vi "Calculate Hold-In Voltage Measurements.vi"(0 "Stage Voltage Section":dbl[](array[numeric]), 5 "Stage.Dwell.Level":dbl, 7 "Active Edge":bool) -> (4 "Max Stage":dbl, 6 "Min Stage":dbl, 10 "Avg Max Stage":dbl, 15 "Avg Min Stage":dbl)   [LabVIEW 2019, in "Fuel Injector Analysis Addon Engine.lvlib"]
uses:
  Fuel Injector Analysis Addon Engine.lvlib
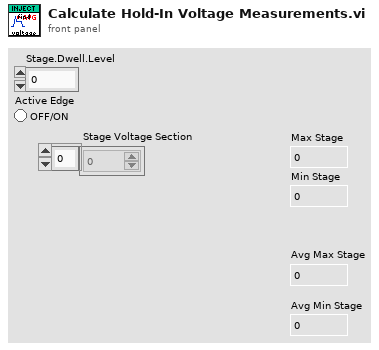
[diagram p1: front panel]
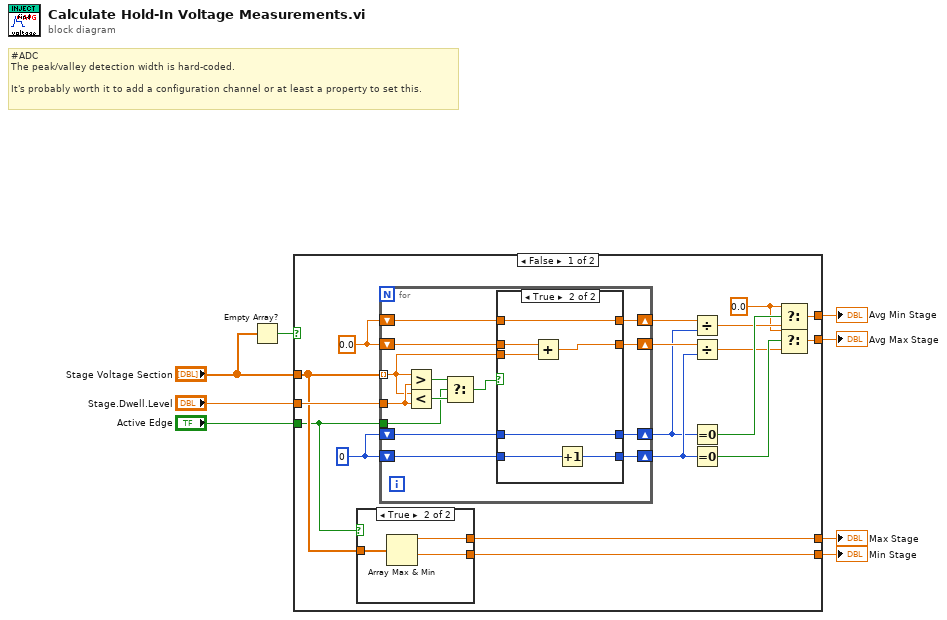
[diagram p0: block diagram]
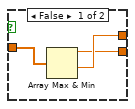
[diagram p2: hidden frame]
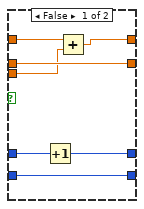
[diagram p3: hidden frame]
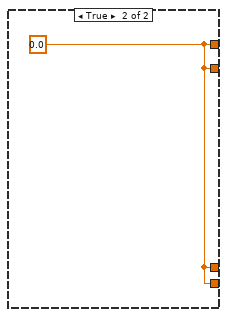
[diagram p4: hidden frame]
diagram:
  # "#ADC \nThe peak/valley detection width is hard-coded.\n\nIt's probably worth it to add a configuration channel or at least a property to set this."
  n1 = Empty Array?(array="Stage Voltage Section") -> (empty?=w2:bool)
  n2 = case shown="False" w2 {
    tunnel: [w26 w61] -> w8
    tunnel: [w25 w61] -> w7
    tunnel: "Stage.Dwell.Level" -> [w20 _]
    tunnel: [w14 w61] -> w5
    tunnel: [w12 w61] -> w4
    tunnel: "Stage Voltage Section" -> [w10 _]
    tunnel: "Active Edge" -> [w9 _]
    frame False {
      w11 = 0.0 ("t")
      w21 = 0
      w23 = 0.0
      n3 = case shown="True" w9 {
        tunnel: [w28 w32] -> w26
        tunnel: [w27 w31] -> w25
        tunnel: w10 -> [w29 w30]
        frame False {
          n4 = Array Max & Min(array=w29) -> (max value=w27:dbl, min value=w28:dbl)  [unwired: 2 out]
        }
        frame True {
          n5 = Array Max & Min(array=w30) -> (max value=w32:dbl, min value=w31:dbl)  [unwired: 2 out]
        }
      }
      n6 = for {
        tunnel: w10 -> [w37] mode=indexing
        tunnel: w20 -> [w38]
        shift-right: [w45] -> w24
        shift-left: w23 -> [w46]
        shift-right: [w43] -> w19
        shift-left: w21 -> [w44]
        shift-right: [w41] -> w18
        shift-left: w21 -> [w42]
        shift-right: [w39] -> w22
        shift-left: w23 -> [w40]
        tunnel: w9 -> [w33]
        n7 = Greater?(x=w37, y=w38) -> (0:w36:bool)
        n8 = Less?(x=w37, y=w38) -> (x < y?=w35:bool)
        n9 = Select(t=w36, s=w33, f=w35) -> (s? t:f=w34:bool)
        n10 = case shown="True" w34 {
          tunnel: w46 -> [w53 w60]
          tunnel: w37 -> [w48 w59]
          tunnel: [w53 w58] -> w45
          tunnel: w44 -> [w52 w57]
          tunnel: [w52 w56] -> w43
          tunnel: w42 -> [w51 w55]
          tunnel: [w50 w55] -> w41
          tunnel: w40 -> [w49 w54]
          tunnel: [w47 w54] -> w39
          frame False {
            n11 = Increment(x=w51) -> (x+1=w50:i32)
            n12 = Add(x=w49, y=w48) -> (x+y=w47:dbl)
          }
          frame True {
            n13 = Add(x=w60, y=w59) -> (x+y=w58:dbl)
            n14 = Increment(x=w57) -> (x+1=w56:i32)
          }
        }
      }
      n15 = Divide(x=w22, y=w18) -> (x/y=w13:dbl)
      n16 = Divide(x=w24, y=w19) -> (x/y=w15:dbl)
      n17 = Equal To 0?(x=w18) -> (x = 0?=w16:bool)
      n18 = Equal To 0?(x=w19) -> (x = 0?=w17:bool)
      n19 = Select(t=w11, s=w16, f=w13) -> (s? t:f=w12:dbl)
      n20 = Select(t=w11, s=w17, f=w15) -> (s? t:f=w14:dbl)
    }
    frame True {
      w61 = 0.0 ("mean")
    }
  }
  "Avg Max Stage" <- w5
  "Max Stage" <- w8
  "Min Stage" <- w7
  "Avg Min Stage" <- w4
